vi "Omron TCP FINS-Handshaking Respond Check.vi"(8 "error in":errorcluster, 11 "Buffer Data In":T1={"Connection ID"=refnum, "Command Code"=enum."Memory area read", "Command String"="", "Read Bytes"=0, "Response String"="FINS\u0000\u0000\u0000\u0010\u0000\u0000\u0000\u0001\u0000\u0000\u0000\u0000\u0000\u0000\u0000›\u0000\u0000\u0000\u0002", "Server Node"=0, "Client Node"=0, "Unit Number"=0}) -> (0 "error out":errorcluster, 3 "Buffer Data Out":T1)   [LabVIEW 2016]
uses:
  Data Def/Omron TCP FINS-Buffer Data.ctl
  Data Def/Omron TCP FINS-Command Code.ctl
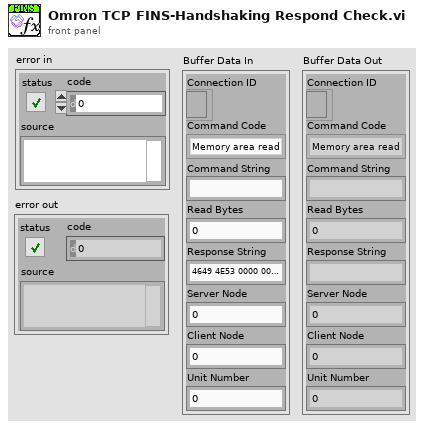
[diagram p1: front panel]
types:
  T1 = typedef "Omron TCP FINS-Buffer Data.ctl" = cluster{"Connection ID":refnum<k5>, "Command Code":T2, "Command String":string, "Read Bytes":i32, "Response String":string, "Server Node":u8, "Client Node":u8, "Unit Number":u8}
  T2 = typedef "Omron TCP FINS-Command Code.ctl" = enum16{"Memory area read", "Memory area write"}
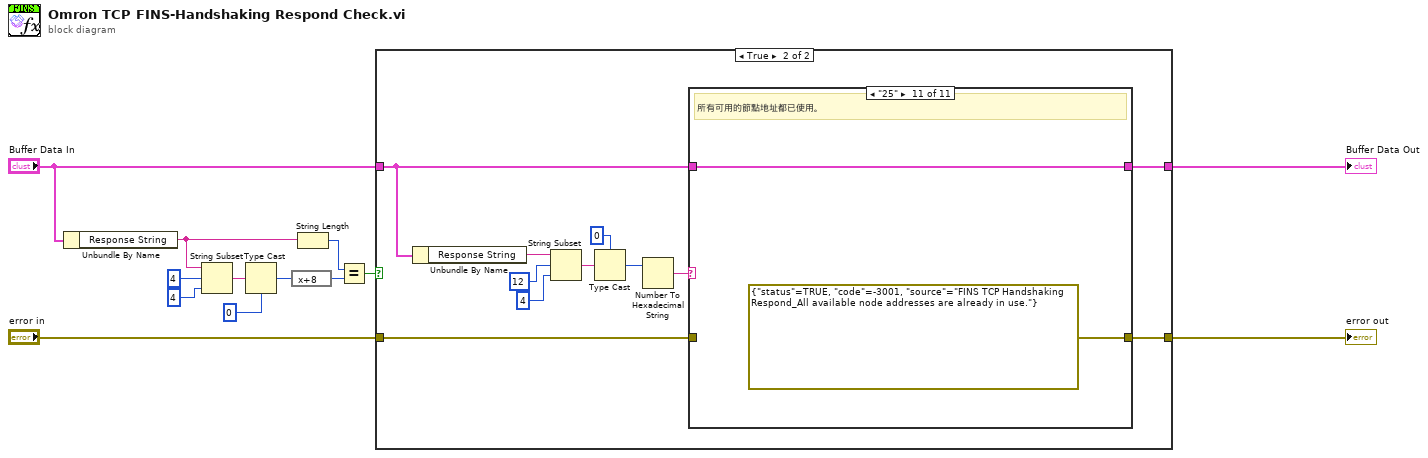
[diagram p0: block diagram]
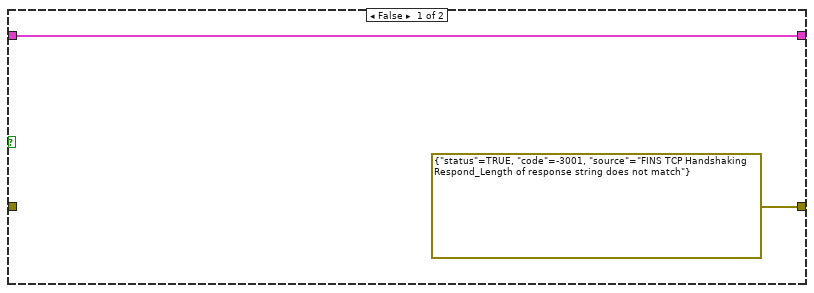
[diagram p2: hidden frame]
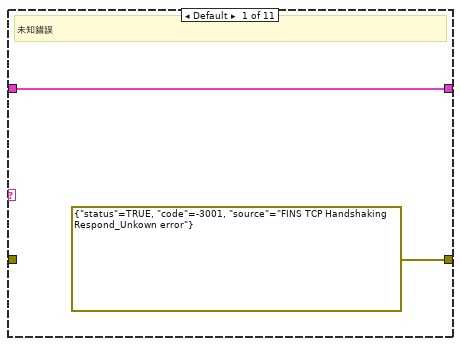
[diagram p3: hidden frame]
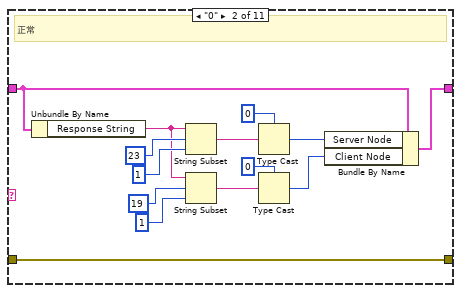
[diagram p4: hidden frame]
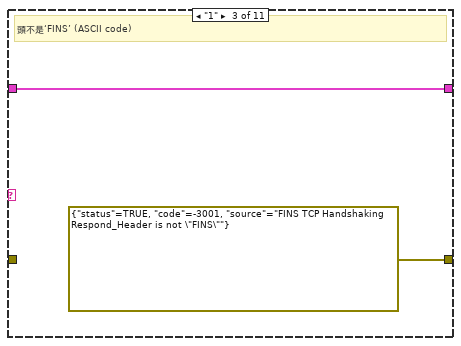
[diagram p5: hidden frame]
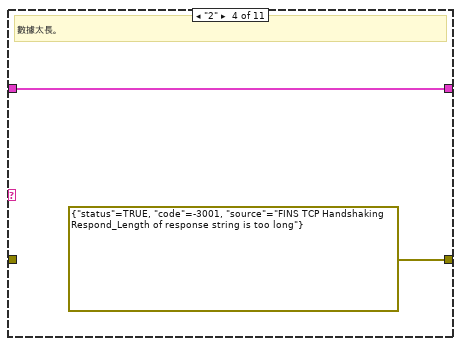
[diagram p6: hidden frame]
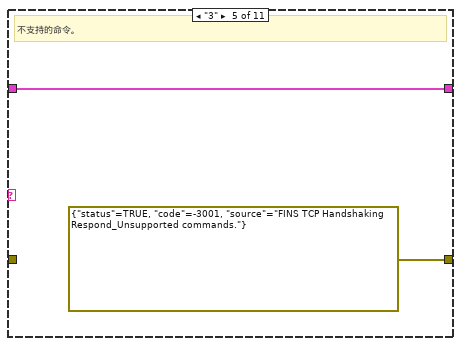
[diagram p7: hidden frame]
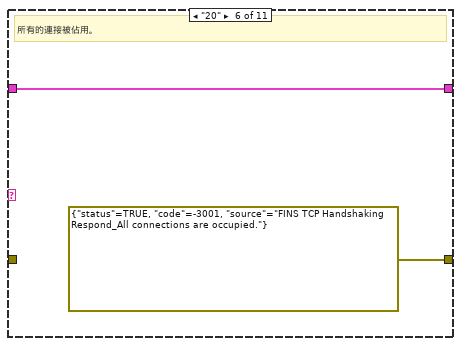
[diagram p8: hidden frame]
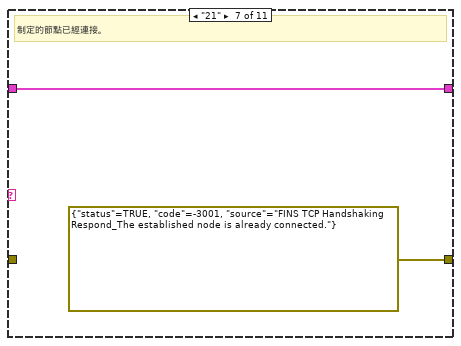
[diagram p9: hidden frame]
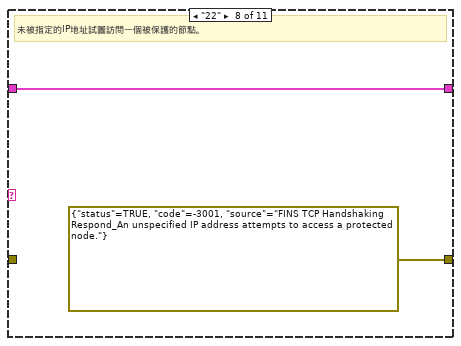
[diagram p10: hidden frame]
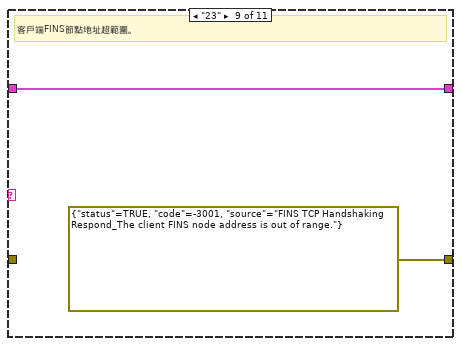
[diagram p11: hidden frame]
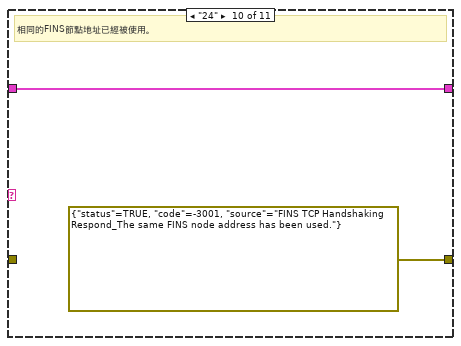
[diagram p12: hidden frame]
diagram:
  n1 = Unbundle By Name("Buffer Data In") -> ("Response String"=w3:string)
  n2 = String Subset(string=w3, offset (0)=4, length (rest)=4 ("length (rest)")) -> (substring=w8:string)
  n3 = Type Cast(type=0, x=w8) -> (*(type *) &x=w2:i32)
  n4 = expression code="x+8"(w2) -> (w1:i32)
  n5 = String Length(string=w3) -> (length=w13:i32)
  n6 = Equal?(x=w13, y=w1) -> (x = y?=w12:bool)
  n7 = case shown="True" w12 {
    tunnel: "Buffer Data In" -> [w15 w18]
    tunnel: "error in" -> [_ w19]
    tunnel: [w15 w17] -> w9
    tunnel: [errorcluster {"status"=TRUE, "code"=-3001, "source"="FINS TCP Handshaking Respond_Length of response string does not match"} ("error in") w16] -> w10
    frame False {
    }
    frame True {
      n8 = Unbundle By Name(w18) -> ("Response String"=w26:string)
      n9 = String Subset(string=w26, offset (0)=12, length (rest)=4 ("length (rest)")) -> (substring=w21:string)
      n10 = Type Cast(type=0, x=w21) -> (*(type *) &x=w23:i32)
      n11 = Number To Hexadecimal String(2:w23) -> (0:w20:string)  [unwired: 1 in]
      n12 = case shown="\"25\"" w20 {
        tunnel: w19 -> [_ w42 _ _ _ _ _ _ _ _ _]
        tunnel: w18 -> [w28 w37 w44 w46 w48 w50 w52 w54 w56 w58 w60]
        tunnel: [w28 w35 w44 w46 w48 w50 w52 w54 w56 w58 w60] -> w17
        tunnel: [errorcluster {"status"=TRUE, "code"=-3001, "source"="FINS TCP Handshaking Respond_Unkown error"} ("error in") w42 errorcluster {"status"=TRUE, "code"=-3001, "source"="FINS TCP Handshaking Respond_Header is not \"FINS\""} ("error in") errorcluster {"status"=TRUE, "code"=-3001, "source"="FINS TCP Handshaking Respond_Length of response string is too long"} ("error in") errorcluster {"status"=TRUE, "code"=-3001, "source"="FINS TCP Handshaking Respond_Unsupported commands."} ("error in") errorcluster {"status"=TRUE, "code"=-3001, "source"="FINS TCP Handshaking Respond_All connections are occupied."} ("error in") errorcluster {"status"=TRUE, "code"=-3001, "source"="FINS TCP Handshaking Respond_The established node is already connected."} ("error in") errorcluster {"status"=TRUE, "code"=-3001, "source"="FINS TCP Handshaking Respond_An unspecified IP address attempts to access a protected node."} ("error in") errorcluster {"status"=TRUE, "code"=-3001, "source"="FINS TCP Handshaking Respond_The client FINS node address is out of range."} ("error in") errorcluster {"status"=TRUE, "code"=-3001, "source"="FINS TCP Handshaking Respond_The same FINS node address has been used."} ("error in") errorcluster {"status"=TRUE, "code"=-3001, "source"="FINS TCP Handshaking Respond_All available node addresses are already in use."} ("error in")] -> w16
        frame Default {
          # "未知錯誤"
        }
        frame "0" {
          # "正常"
          n13 = Unbundle By Name(w37) -> ("Response String"=w33:string)
          n14 = String Subset(string=w33, offset (0)=23, length (rest)=1 ("length (rest)")) -> (substring=w39:string)
          n15 = String Subset(string=w33, offset (0)=19, length (rest)=1 ("length (rest)")) -> (substring=w30:string)
          n16 = Type Cast(type=u8 0, x=w39) -> (*(type *) &x=w36:u8)
          n17 = Type Cast(type=u8 0, x=w30) -> (*(type *) &x=w29:u8)
          n18 = Bundle By Name(cluster=w37, "Server Node"=w36, "Client Node"=w29) -> (w35:T1)
        }
        frame "1" {
          # "頭不是‘FINS’ (ASCII code)"
        }
        frame "2" {
          # "數據太長。"
        }
        frame "3" {
          # "不支持的命令。"
        }
        frame "20" {
          # "所有的連接被佔用。"
        }
        frame "21" {
          # "制定的節點已經連接。"
        }
        frame "22" {
          # "未被指定的IP地址試圖訪問一個被保護的節點。"
        }
        frame "23" {
          # "客戶端FINS節點地址超範圍。"
        }
        frame "24" {
          # "相同的FINS節點地址已經被使用。"
        }
        frame "25" {
          # "所有可用的節點地址都已使用。"
        }
      }
    }
  }
  "error out" <- w10
  "Buffer Data Out" <- w9
